vi "Write.Initialize.vi"(8 "error in":errorcluster, 10 "VS Engine Interface":refnum<class "VS Engine Interface.lvclass">, 11 "Settings":cluster{"Refs":T1[], "Values":dbl[]} {"Refs" format="%.0x"}) -> (0 "error out":errorcluster, 3 "Write out":refnum<class "Write.lvclass">)   [LabVIEW 2024, in "VS Plugin Inline Async API.lvlib" / "Write.lvclass"]
uses:
  Write.lvclass
  Write.lvclass/Write.ctl
  <vilib>/NI VeriStand/Custom Device API/Data Reference.ctl
  <vilib>/NI VeriStand/Custom Device API/Custom Device API.lvlib
  VS Engine Abstraction/VS Engine Interface/VS Engine Interface.lvclass
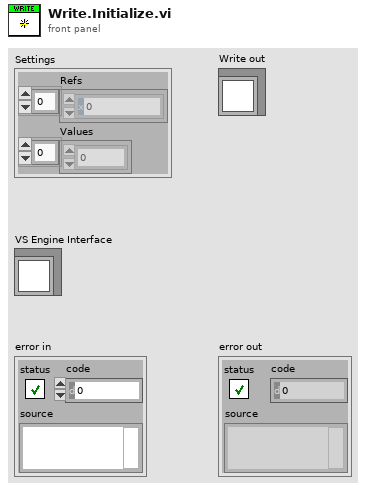
[diagram p1: front panel]
types:
  T1 = typedef "Custom Device API.lvlib/Data Reference.ctl" = i32
  T2 = cluster{"read mode":enum16{"polling", "blocking"}, "write mode":enum16{"polling", "blocking"}}
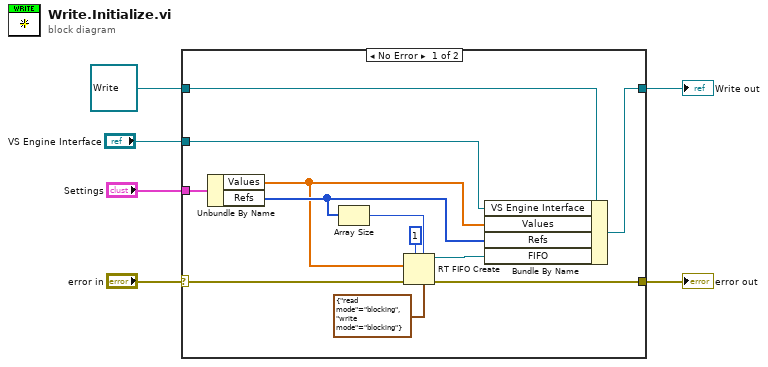
[diagram p0: block diagram]
diagram:
  n1 = case shown="No Error" "error in" {
    selector: "error in" -> [w17 w20]
    tunnel: [w18 w20] -> w5
    tunnel: refnum<class "Write.lvclass"> refnum ("Write in") -> [w12 w19]
    tunnel: [w11 w19] -> w2
    tunnel: "Settings" -> [w10 _]
    tunnel: "VS Engine Interface" -> [w7 _]
    frame No Error {
      n2 = Unbundle By Name(w10) -> ("Values"=w8:dbl[], "Refs"=w9:T1[])
      n3 = Array Size(array=w9) -> (size(s)=w14:i32)
      n4 = RT FIFO Create(1:w8, 3:w17, 4:u32 1 ("size (10)"), 6:w14, 7:T2 {"read mode"=enum."blocking", "write mode"=enum."blocking"} ("r/w modes (polling,polling)")) -> (8:w16:refnum<k33>, 11:w18:errorcluster)  [unwired: 3 in, 1 out]
      n5 = Bundle By Name(cluster=w12, "VS Engine Interface"=w7, "Values"=w8, "Refs"=w9, "FIFO"=w16) -> (w11:refnum<class "Write.lvclass">)
    }
    frame Error {
    }
  }
  "error out" <- w5
  "Write out" <- w2
